vi "Cluster to Variant Attributes.vi"(8 "error in (no error)":errorcluster, 11 "Cluster":variant) -> (0 "error out":errorcluster, 3 "Variant":variant)   [LabVIEW 2020, in "ORM_API.lvlib"]
uses:
  ORM_API.lvlib
  <userlib>/_OpenG.lib/lvdata/lvdata.llb/openg_variant.lvlib
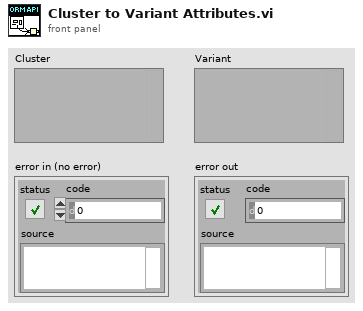
[diagram p1: front panel]
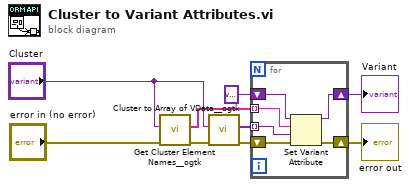
[diagram p0: block diagram]
diagram:
  n1 = call <userlib>:"Get Cluster Element Names__ogtk.vi"("error in (no error)"="error in (no error)", "Cluster"="Cluster") -> ("error out"=w6:errorcluster, "Element Names"=w2:string[])  [unwired: 8 in]
  n2 = call <userlib>:"Cluster to Array of VData__ogtk.vi"("error in (no error)"=w6, "Cluster"="Cluster") -> ("error out"=w8:errorcluster, "Array of VData"=w3:variant[])  [unwired: 8 in]
  n3 = for {
    tunnel: w2 -> [w15] mode=indexing
    tunnel: w3 -> [w14] mode=indexing
    shift-right: [w12] -> w5
    shift-left: variant ("Variant") -> [w13]
    shift-right: [w10] -> w9
    shift-left: w8 -> [w11]
    n4 = Set Variant Attribute(Variant=w13, name=w15, value=w14, error in=w11) -> (Variant out=w12:variant, error out=w10:errorcluster)  [unwired: 1 out]
  }
  "error out" <- w9
  "Variant" <- w5
